vi "Ustawienie ostatniego położenia na podstawie odległości od punktu startowego.vi"(9 "Długość piksela w metrach":dbl, 10 "Odległość od startu [m]":cluster{"X [m]":dbl, "Y [m]":dbl}, 11 "Poł. startowe":cluster{"Piksel x":i32, "Piksel y":i32}) -> (3 "Ostatnie położenie robota":cluster{"Pixel x":i16, "Pixel y":i16})   [LabVIEW 2012, in "Biblioteka moduł map v3.lvlib" / "Obsługa grafiki mapy.lvlib"]
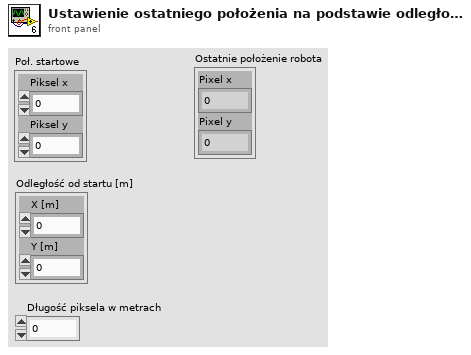
[diagram p1: front panel]
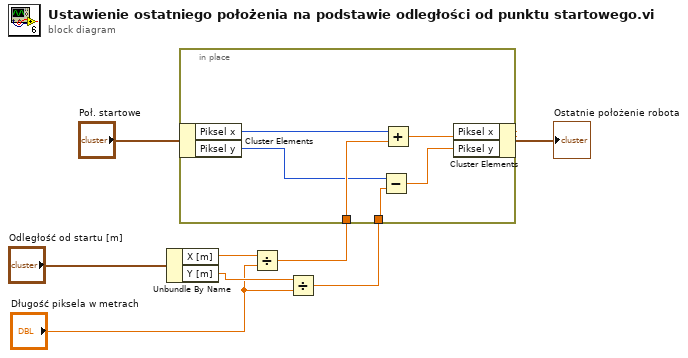
[diagram p0: block diagram]
diagram:
  n1 = Unbundle By Name("Odległość od startu [m]") -> ("X [m]"=w6:dbl, "Y [m]"=w5:dbl)
  n2 = Divide(x=w6, y="Długość piksela w metrach") -> (x/y=w3:dbl)
  n3 = Divide(x=w5, y="Długość piksela w metrach") -> (x/y=w2:dbl)
  n4 = in-place {
    in-place-border: w3 -> [w14]
    in-place-border: w2 -> [w11]
    n5 = in-place-cluster #1("Poł. startowe") -> ("Piksel x"=w13:i32, "Piksel y"=w12:i32)
    n6 = Subtract(x=w12, y=w11) -> (x-y=w9:dbl)
    n7 = Add(x=w13, y=w14) -> (x+y=w10:dbl)
    n8 = in-place-cluster #1("Piksel x"=w10, "Piksel y"=w9) -> (→"Ostatnie położenie robota":cluster{"Piksel x":i32, "Piksel y":i32})
  }
